vi "readFromXML.vi"(8 "error in (no error)":errorcluster, 10 "XML in":string, 11 "RotCurrentWrap in":refnum<class "RotCurrentWrap.lvclass">) -> (0 "error out":errorcluster, 3 "RotCurrentWrap out":refnum<class "RotCurrentWrap.lvclass">)   [LabVIEW 2014, in "TCSDataDefinitions.lvlib" / "TCSCommand.lvlib" / "CableWrapCommands.lvlib" / "RotCurrentWrap.lvclass"]
uses:
  RotCurrentWrap.lvclass
  CableWrapCommands/CableWrapCommands.lvclass
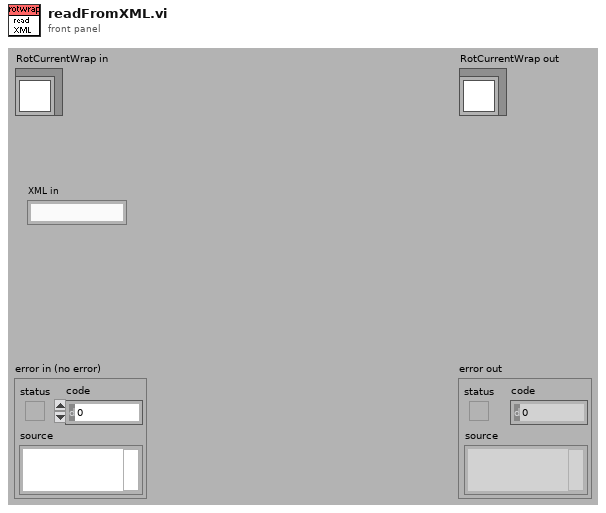
[diagram p1: front panel]
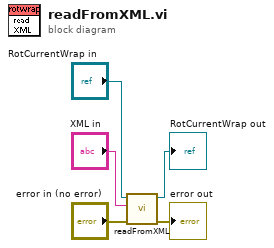
[diagram p0: block diagram]
diagram:
  n1 = call-parent "readFromXML.vi"("error in (no error)"="error in (no error)", "XML in"="XML in", "CableWrapCommands in"="RotCurrentWrap in") -> ("error out"=→"error out":errorcluster, "CableWrapCommands out"=→"RotCurrentWrap out":refnum<class "RotCurrentWrap.lvclass">)  [unwired: 7 out]
